vi "CMS Contol Console.vi"() -> ()   [LabVIEW 2019]
uses:
  <vilib>/Instr/_visa.llb/VISA Configure Serial Port (Instr).vi
panel:
  in  "Boolean 3":bool
  in  "Boolean":bool
  in  "COM PORT":string(combo)
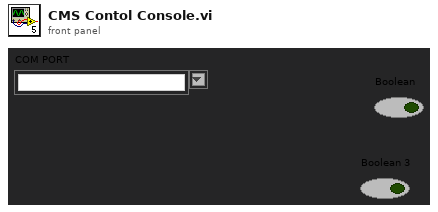
[diagram p1: front panel]
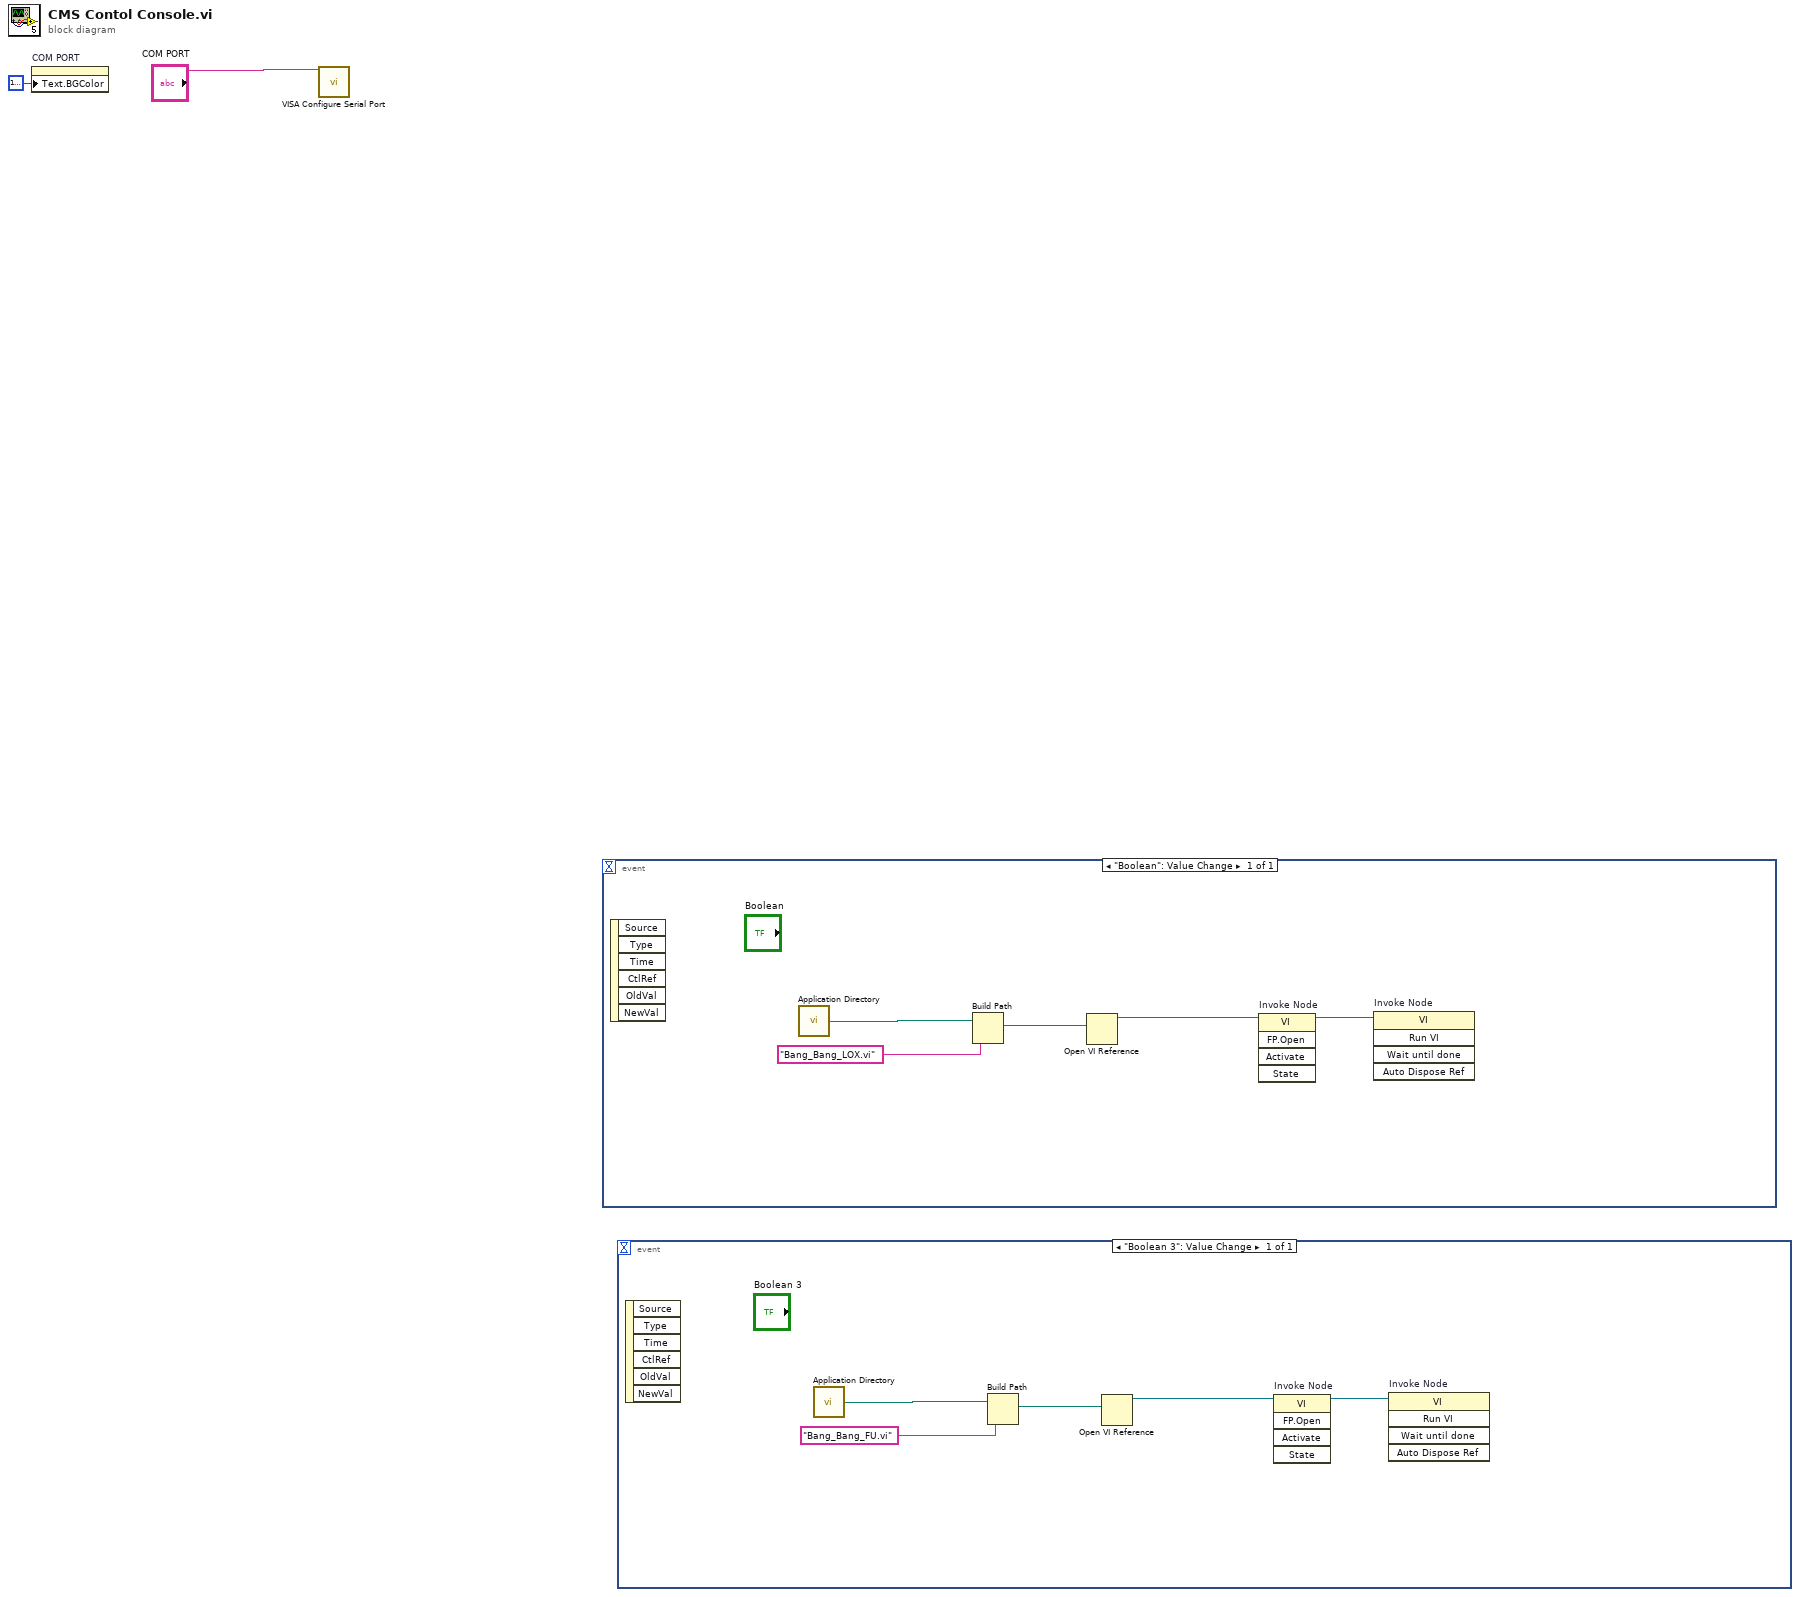
[diagram p0: block diagram]
diagram:
  n1 = property on="COM PORT" class="CmbBox"("Text.BGColor"=u32 16777226 ("Text.Text Colors:BG Color")) -> ()  [unwired: 2 in, 2 out]
  n2 = call-poly "VISA Configure Serial Port"("VISA resource name"="COM PORT") -> ()  [unwired: 13 in, 2 out]
  n3 = event shown="[0] \"Boolean\": Value Change" {
    selector: _ -> [_]
    dyn-events: _ -> [_]
    timeout: _ -> [_]
    event "Boolean": Value Change {
      n4 = event-data() -> ()  [unwired: 1 in, 6 out]
      n5 = call <vilib>:"Application Directory.vi"() -> ("Application Directory"=w4:path)
      n6 = Build Path(base path=w4, name or relative path="Bang_Bang_LOX.vi") -> (appended path=w5:path)
      n7 = Open VI Reference(vi path=w5) -> (vi reference=w6:refnum<vi>)  [unwired: 5 in, 1 out]
      n8 = invoke on="Invoke Node" class="VI" method="FP.Open"(reference=w6) -> (reference out=w7:refnum<vi>)  [unwired: 4 in, 4 out]
      n9 = invoke on="Invoke Node" class="VI" method="Run VI"(reference=w7) -> ()  [unwired: 4 in, 5 out]
    }
  }
  n10 = event shown="[0] \"Boolean 3\": Value Change" {
    selector: _ -> [_]
    dyn-events: _ -> [_]
    timeout: _ -> [_]
    event "Boolean 3": Value Change {
      n11 = event-data() -> ()  [unwired: 1 in, 6 out]
      n12 = call <vilib>:"Application Directory.vi"() -> ("Application Directory"=w9:path)
      n13 = Build Path(base path=w9, name or relative path="Bang_Bang_FU.vi") -> (appended path=w10:path)
      n14 = Open VI Reference(vi path=w10) -> (vi reference=w11:refnum<vi>)  [unwired: 5 in, 1 out]
      n15 = invoke on="Invoke Node" class="VI" method="FP.Open"(reference=w11) -> (reference out=w12:refnum<vi>)  [unwired: 4 in, 4 out]
      n16 = invoke on="Invoke Node" class="VI" method="Run VI"(reference=w12) -> ()  [unwired: 4 in, 5 out]
    }
  }
